vi "ESP301GroupMove.vi"(0 "VISA resource name":refnum<visa-resource-name>, 1 "Slave Axis":i32, 5 "Group Cluster":T1, 7 "MaxMotion":dbl, 9 "Master Axis":i32, 11 "error in":errorcluster, 12 "Reduction":dbl) -> (4 "VISA resource name out":refnum<visa-resource-name>, 10 "error out":errorcluster)   [LabVIEW 2011]
uses:
  <instrlib>/Newport ESP301/Newport ESP301.lvlib
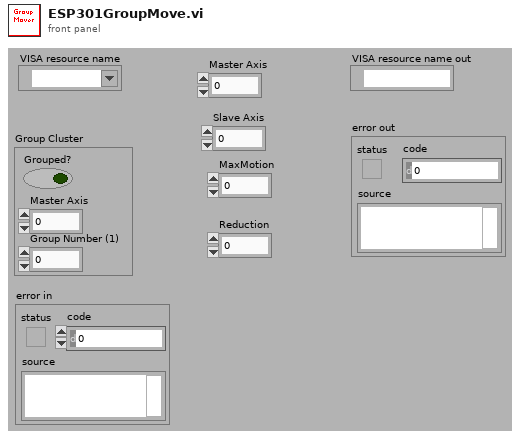
[diagram p1: front panel]
types:
  T1 = cluster{"Grouped?":bool, "Master Axis":i32, "Group Number (1)":i32}
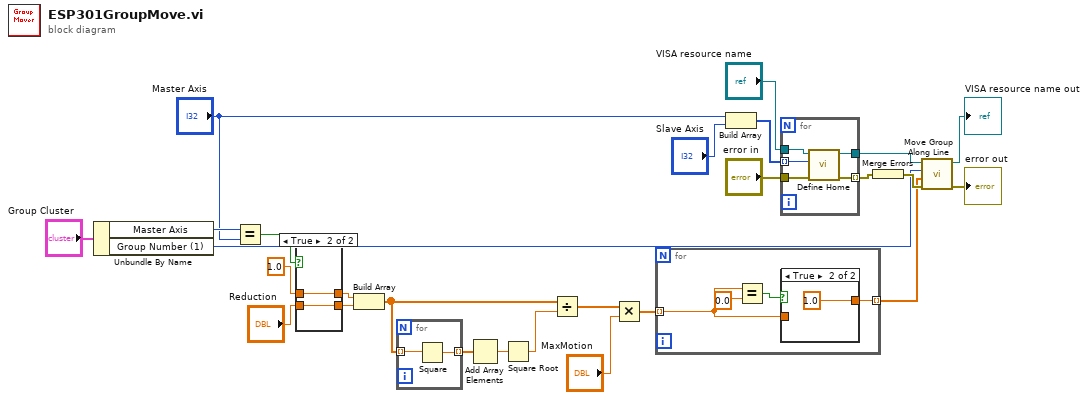
[diagram p0: block diagram]
diagram:
  n1 = Unbundle By Name("Group Cluster") -> ("Master Axis"=w14:i32, "Group Number (1)"=w4:i32)
  n2 = Equal?(x=w14, y="Master Axis") -> (x = y?=w21:bool)
  n3 = case shown="True" w21 {
    tunnel: 1.0 -> [w28 w30]
    tunnel: "Reduction" -> [w27 w29]
    tunnel: [w27 w30] -> w19
    tunnel: [w28 w29] -> w20
    frame False {
    }
    frame True {
    }
  }
  n4 = Build Array(w19, w20) -> (w25:dbl[])
  n5 = for {
    tunnel: w25 -> [w32] mode=indexing
    tunnel: [w31] -> w23 mode=indexing
    n6 = Square(x=w32) -> (x^2=w31:dbl)
  }
  n7 = Add Array Elements(numeric array=w23) -> (sum=w24:dbl)
  n8 = Square Root(x=w24) -> (sqrt(x)=w3:dbl)
  n9 = Divide(x=w25, y=w3) -> (x/y=w2:dbl[])
  n10 = Multiply(x=w2, y="MaxMotion") -> (x*y=w1:dbl[])
  n11 = for {
    tunnel: w1 -> [w34] mode=indexing
    tunnel: [w33] -> w5 mode=indexing
    n12 = Equal?(x=w34, y=0.0) -> (x = y?=w35:bool)
    n13 = case shown="True" w35 {
      tunnel: w34 -> [w37 _]
      tunnel: [w37 1.0 ("y")] -> w33
      frame False {
      }
      frame True {
      }
    }
  }
  n14 = Build Array("Master Axis", "Slave Axis") -> (w11:i32[])
  n15 = for {
    tunnel: w11 -> [w43] mode=indexing
    tunnel: "VISA resource name" -> [w42]
    tunnel: "error in" -> [w41]
    tunnel: [w40] -> w8 mode=indexing
    tunnel: [w39] -> w7
    n16 = call <instrlib>:"Define Home.vi"("error in (no error)"=w41, "Axis (1)"=w43, "VISA resource name"=w42) -> ("error out"=w40:errorcluster, "VISA resource name out"=w39:refnum<visa-resource-name>)  [unwired: 3 in]
  }
  n17 = Merge Errors(w8) -> (w6:errorcluster)
  n18 = call <instrlib>:"Move Group Along Line.vi"("error in (no error)"=w6, "Position (0 units)"=w5, "Group Number (1)"=w4, "VISA resource name"=w7) -> ("error out"=→"error out":errorcluster, "VISA resource name out"=→"VISA resource name out":refnum<visa-resource-name>)  [unwired: 2 in]
